vi "Read Analogue.vi"(8 "error in (no error)":errorcluster, 11 "PS in":refnum<class "Keysight 6700C.lvclass">) -> (0 "error out":errorcluster, 2 "Measurements":dbl, 3 "PS out":refnum<class "Keysight 6700C.lvclass">)   [LabVIEW 2019, in "Concrete.lvlib" / "Keysight 6700C.lvclass"]
uses:
  Keysight 6700C.lvclass
  Keysight 6700C.lvclass/Keysight 6700C.ctl
  Harware Abstraction/Analog out/Analog out.lvclass
  <instrlib>/Agilent N6700/Agilent N6700 Series.lvlib
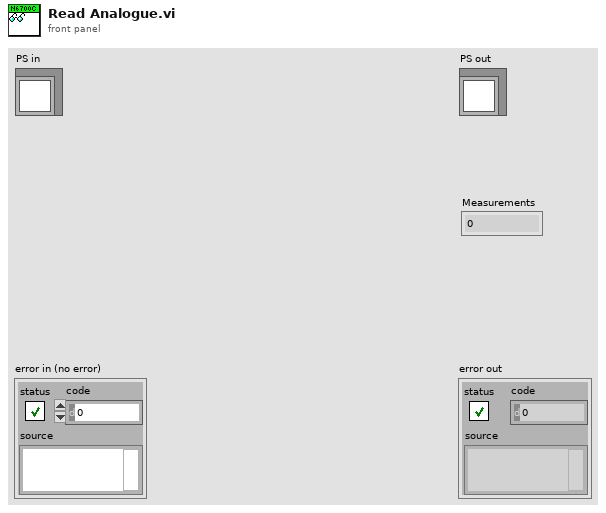
[diagram p1: front panel]
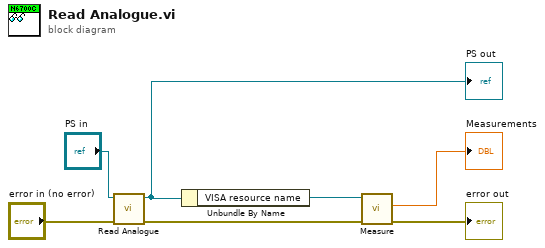
[diagram p0: block diagram]
diagram:
  n1 = call-parent "Read Analogue.vi"("error in (no error)"="error in (no error)", "Analog out in"="PS in") -> ("error out"=w5:errorcluster, "Analog out out"=w3:refnum<class "Keysight 6700C.lvclass">)  [unwired: 7 in, 1 out]
  "PS out" <- w3
  n2 = Unbundle By Name(w3) -> ("VISA resource name"=w2:refnum<visa-resource-name>)
  n3 = call <instrlib>:"Measure.vi"("error in (no error)"=w5, "VISA resource name"=w2) -> ("error out"=→"error out":errorcluster, "Measurement"=→"Measurements":dbl)  [unwired: 7 in, 1 out]
